vi "Aircraft Main.vi"(8 "error out":errorcluster, 11 "Aircraft Index":u8) -> (0 "error out 2":errorcluster)   [LabVIEW 2014]
uses:
  Application Support/Stop Button/SubVI/Get Stop Button Status.vi
  MAVLink/Commands/MAV_CMD Sub VI/MAV_CMD_COMPONENT_ARM_DISARM.vi
  Controls/Aircraft State.ctl
  Joystick/FGVs/Joystick Input/Method VIs/Get Joystick Input.vi
  Aircraft Information/Sub VI/Get Aircraft System Status.vi
  Aircraft Information/Sub VI/Set Aircraft System Status.vi
  Aircraft Information/Controls/Aircraft RC Data.ctl
  Aircraft Information/Controls/Aircraft Attitude Data.ctl
  Aircraft Information/Controls/Base Mode.ctl
  Aircraft Information/Controls/Drone Information.ctl
  Aircraft Information/Controls/Aircraft Mode.ctl
  Aircraft Information/Controls/Aircraft Sensor Status Data.ctl
  GUI Design/Indicators/Status LED.ctl
  GUI Design/Indicators/Sensor Status LED CLuster.ctl
  Controls/Telemetry Connection Type.ctl
panel:
  in  "Altitude (m)":sgl
  in  "Takeoff":bool
  in  "Main Tab":T1(tab)
  in  "Aircraft State":T2=enum."Initialise"
  out "Aircraft Att Data Out":T3
  out "Aircraft RC Data Out":T4
  out "Control Mode":T5=enum."Stabalise"
  out "Armed/Disarmed":bool
  in  "param_id":string
  in  "Request Param":bool
  in  "Get Message":bool
  in  "Message Rate (hz)":u16=5
  in  "start_stop":bool
  in  "req_stream_id":T6(ring)
  in  "Aircraft Update Rate (Hz)":dbl=30.0
  in  "Release Control":bool
  out "TX Queue State":i32(slide) scale=0.0..50.0
  out "RX Queue State":i32(slide) scale=0.0..50.0
  out "System Status Out":T7 {"Communication Drop Rate (%)" scale=0.0..100.0; "Battery Remaining (%)" scale=0.0..100.0; "CPU Load (%)" scale=0.0..100.0}
  out "Status text":string
  in  "Clear Status Text":bool
  in  "ARM/DISARM":bool
  out "Drone Information Out":T10={"Heart Beat"=FALSE, "Aircraft ID"=0, "Downlink Port"="", "Tag ID"="", "System Status"="", "Base Mode"={"Custom Mode"=FALSE, "Test Enabled"=FALSE, "Autonomous Mode"=FALSE, "Guided Mode"=FALSE, "Stabilization Enabled"=FALSE, "HIL Enabled"=FALSE, "Manual Mode"=FALSE, "Arm"=FALSE}, "Armed/Disarmed"=FALSE, "Battery Voltage"=0.0, "Control Mode"=enum."Stabalise", "Initialisation"=0, "Heart Beat Status"=FALSE, "Uplink Port"="", "UDP connection ID"=refnum, "Connection Type"=enum."Serial", "Mode"="", "UDP IP Address"="", "Mission Uploaded"=FALSE} {"Initialisation" scale=0.0..100.0}
  out "Initialisation Progress":u8(slide) scale=0.0..100.0
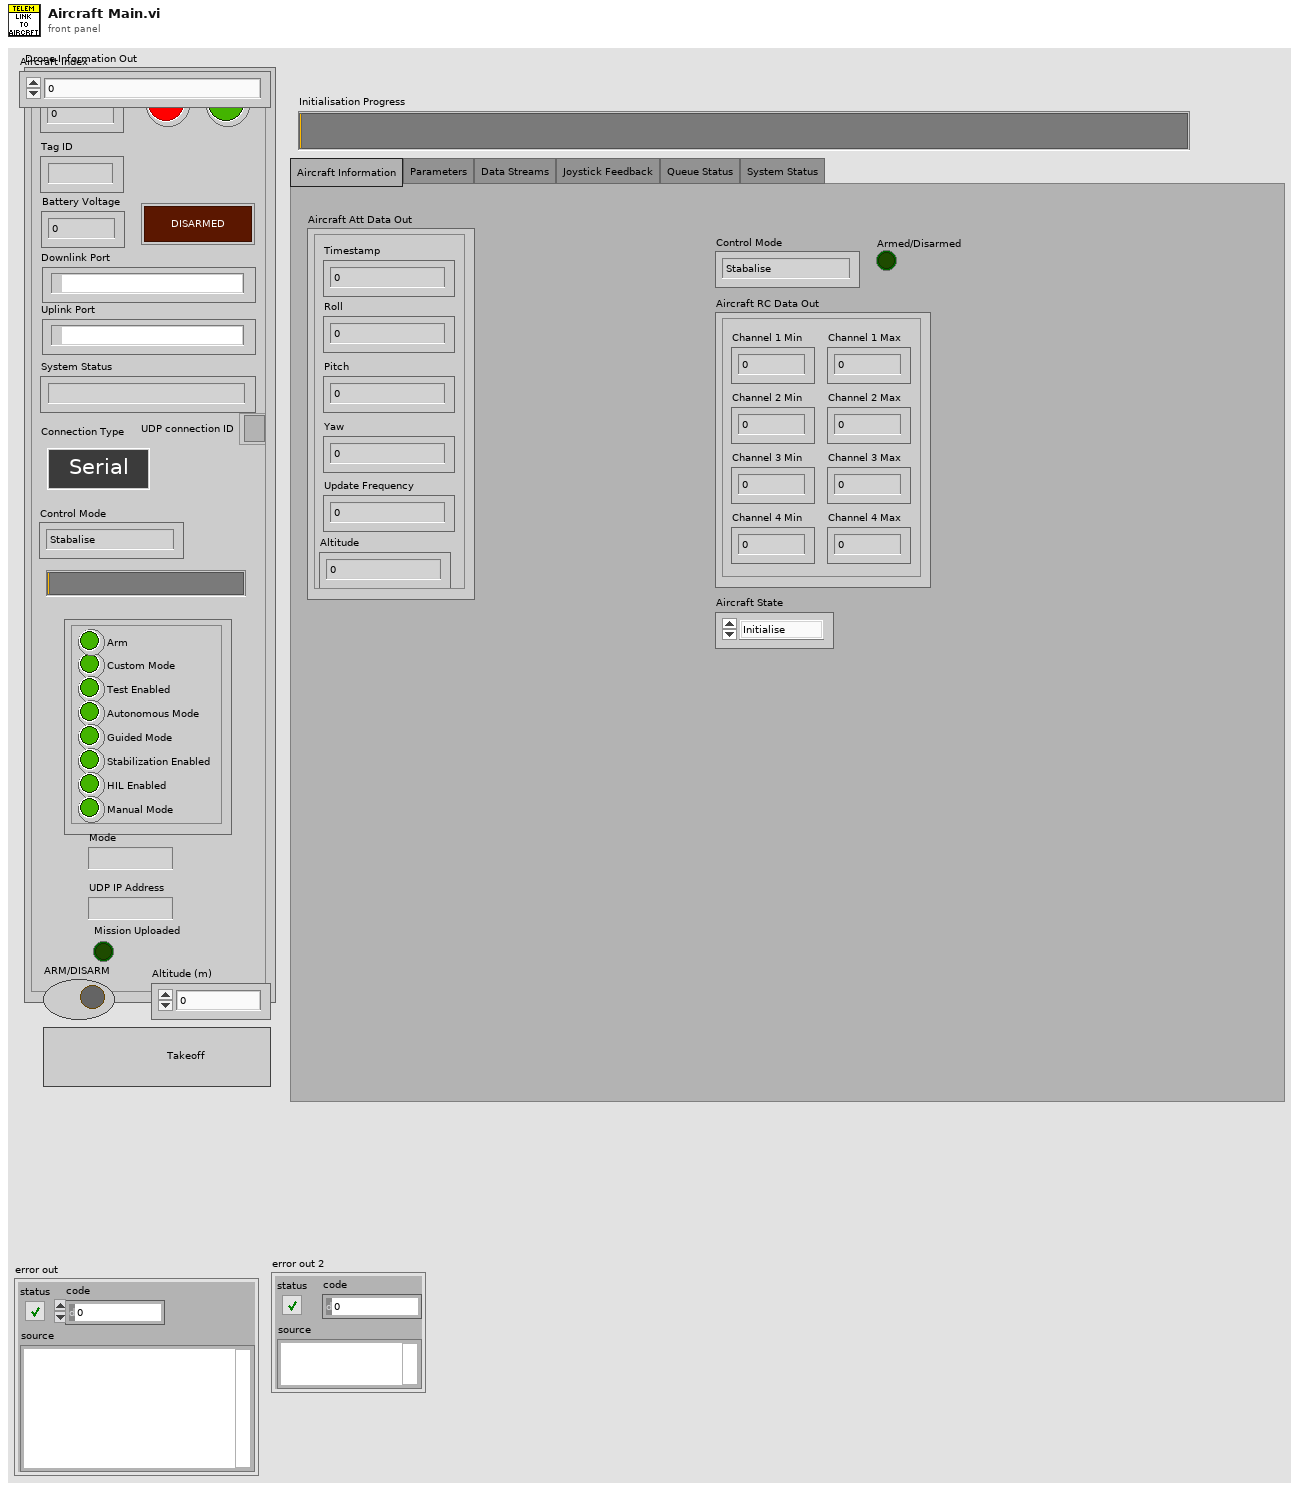
[diagram p1: front panel]
types:
  T1 = enum32{"Aircraft Information", "Parameters", "Data Streams", "Joystick Feedback", "Queue Status", "System Status"}
  T2 = typedef "Aircraft State.ctl" = enum16{"Connected", "Initialise", "Disconnected"}
  T3 = typedef "Aircraft Attitude Data.ctl" = cluster{"Roll":sgl, "Pitch":sgl, "Yaw":sgl, "Timestamp":u32, "Update Frequency":dbl, "Altitude":sgl}
  T4 = typedef "Aircraft RC Data.ctl" = cluster{"Channel 1 Min":i16, "Channel 1 Max":i16, "Channel 2 Min":i16, "Channel 2 Max":i16, "Channel 3 Min":i16, "Channel 3 Max":i16, "Channel 4 Min":i16, "Channel 4 Max":i16}
  T5 = typedef "Aircraft Mode.ctl" = enum16{"Loiter", "Stabalise", "Failsafe", "Emergency Stop"}
  T6 = enum16{"ALL", "RAW_SENSORS", "EXTENDED_STATUS", "RC_CHANNELS", "RAW_CONTROLLER", "POSITION", "EXTRA1", "EXTRA2", "EXTRA3"}
  T7 = typedef "Aircraft Sensor Status Data.ctl" = cluster{"Sensor Status":T8, "CPU Load (%)":dbl, "Battery Voltage (V)":dbl, "Battery Current (A)":dbl, "Battery Remaining (%)":dbl, "Communication Drop Rate (%)":dbl, "Communication Errors (%)":dbl, "Status text":string}
  T8 = typedef "Sensor Status LED CLuster.ctl" = cluster{"3D Gyro":u32, "3D Accel":u32, "3D Mag":u32, "Abs. Pressure":u32, "Diff. Pressure":u32, "GPS":T9, "Optical Flow":u32, "Vision Position":u32, "Laser Position":u32, "External Ground Truth":u32, "Angular Rate Control":u32, "Attitude Stabilisation":u32, "Yaw Position":u32, "Z Altitude Control":u32, "XY Position Control":u32, "Motor Outputs":u32, "RC Receiver":u32, "3D Gyro 2":u32, "3D Accel 2":u32, "3D Mag 2":u32, "Geofence":u32, "AHRS":u32, "Terrain":u32}
  T9 = typedef "Status LED.ctl" = u32
  T10 = typedef "Drone Information.ctl" = cluster{"Heart Beat":bool, "Aircraft ID":u8, "Downlink Port":refnum<visa-resource-name>, "Tag ID":string, "System Status":string, "Base Mode":T11, "Armed/Disarmed":bool, "Battery Voltage":dbl, "Control Mode":T5, "Initialisation":u8, "Heart Beat Status":bool, "Uplink Port":refnum<visa-resource-name>, "UDP connection ID":refnum<k16>, "Connection Type":T12, "Mode":string, "UDP IP Address":string, "Mission Uploaded":bool}
  T11 = typedef "Base Mode.ctl" = cluster{"Custom Mode":bool, "Test Enabled":bool, "Autonomous Mode":bool, "Guided Mode":bool, "Stabilization Enabled":bool, "HIL Enabled":bool, "Manual Mode":bool, "Arm":bool}
  T12 = typedef "Telemetry Connection Type.ctl" = enum16{"Serial", "UDP", "TCP"}
  T13 = typedef "Joystick Input.ctl" = cluster{"Roll (%)":dbl, "Pitch (%)":dbl, "Yaw (%)":dbl, "Throttle (%)":dbl, "Brake":bool, "Emergency Stop":bool, "Arm":bool, "Disarm":bool}
  T14 = cluster{"req_message_rate":u16, "target_system":u8, "target_component":u8, "req_stream_id":enum16{"ALL", "RAW_SENSORS", "EXTENDED_STATUS", "RC_CHANNELS", "RAW_CONTROLLER", "POSITION", "EXTRA1", "EXTRA2", "EXTRA3"}, "start_stop":bool}
  T15 = cluster{"chan1_raw":u16, "chan2_raw":u16, "chan3_raw":u16, "chan4_raw":u16, "chan5_raw":u16, "chan6_raw":u16, "chan7_raw":u16, "chan8_raw":u16, "target_system":u8, "target_component":u8}
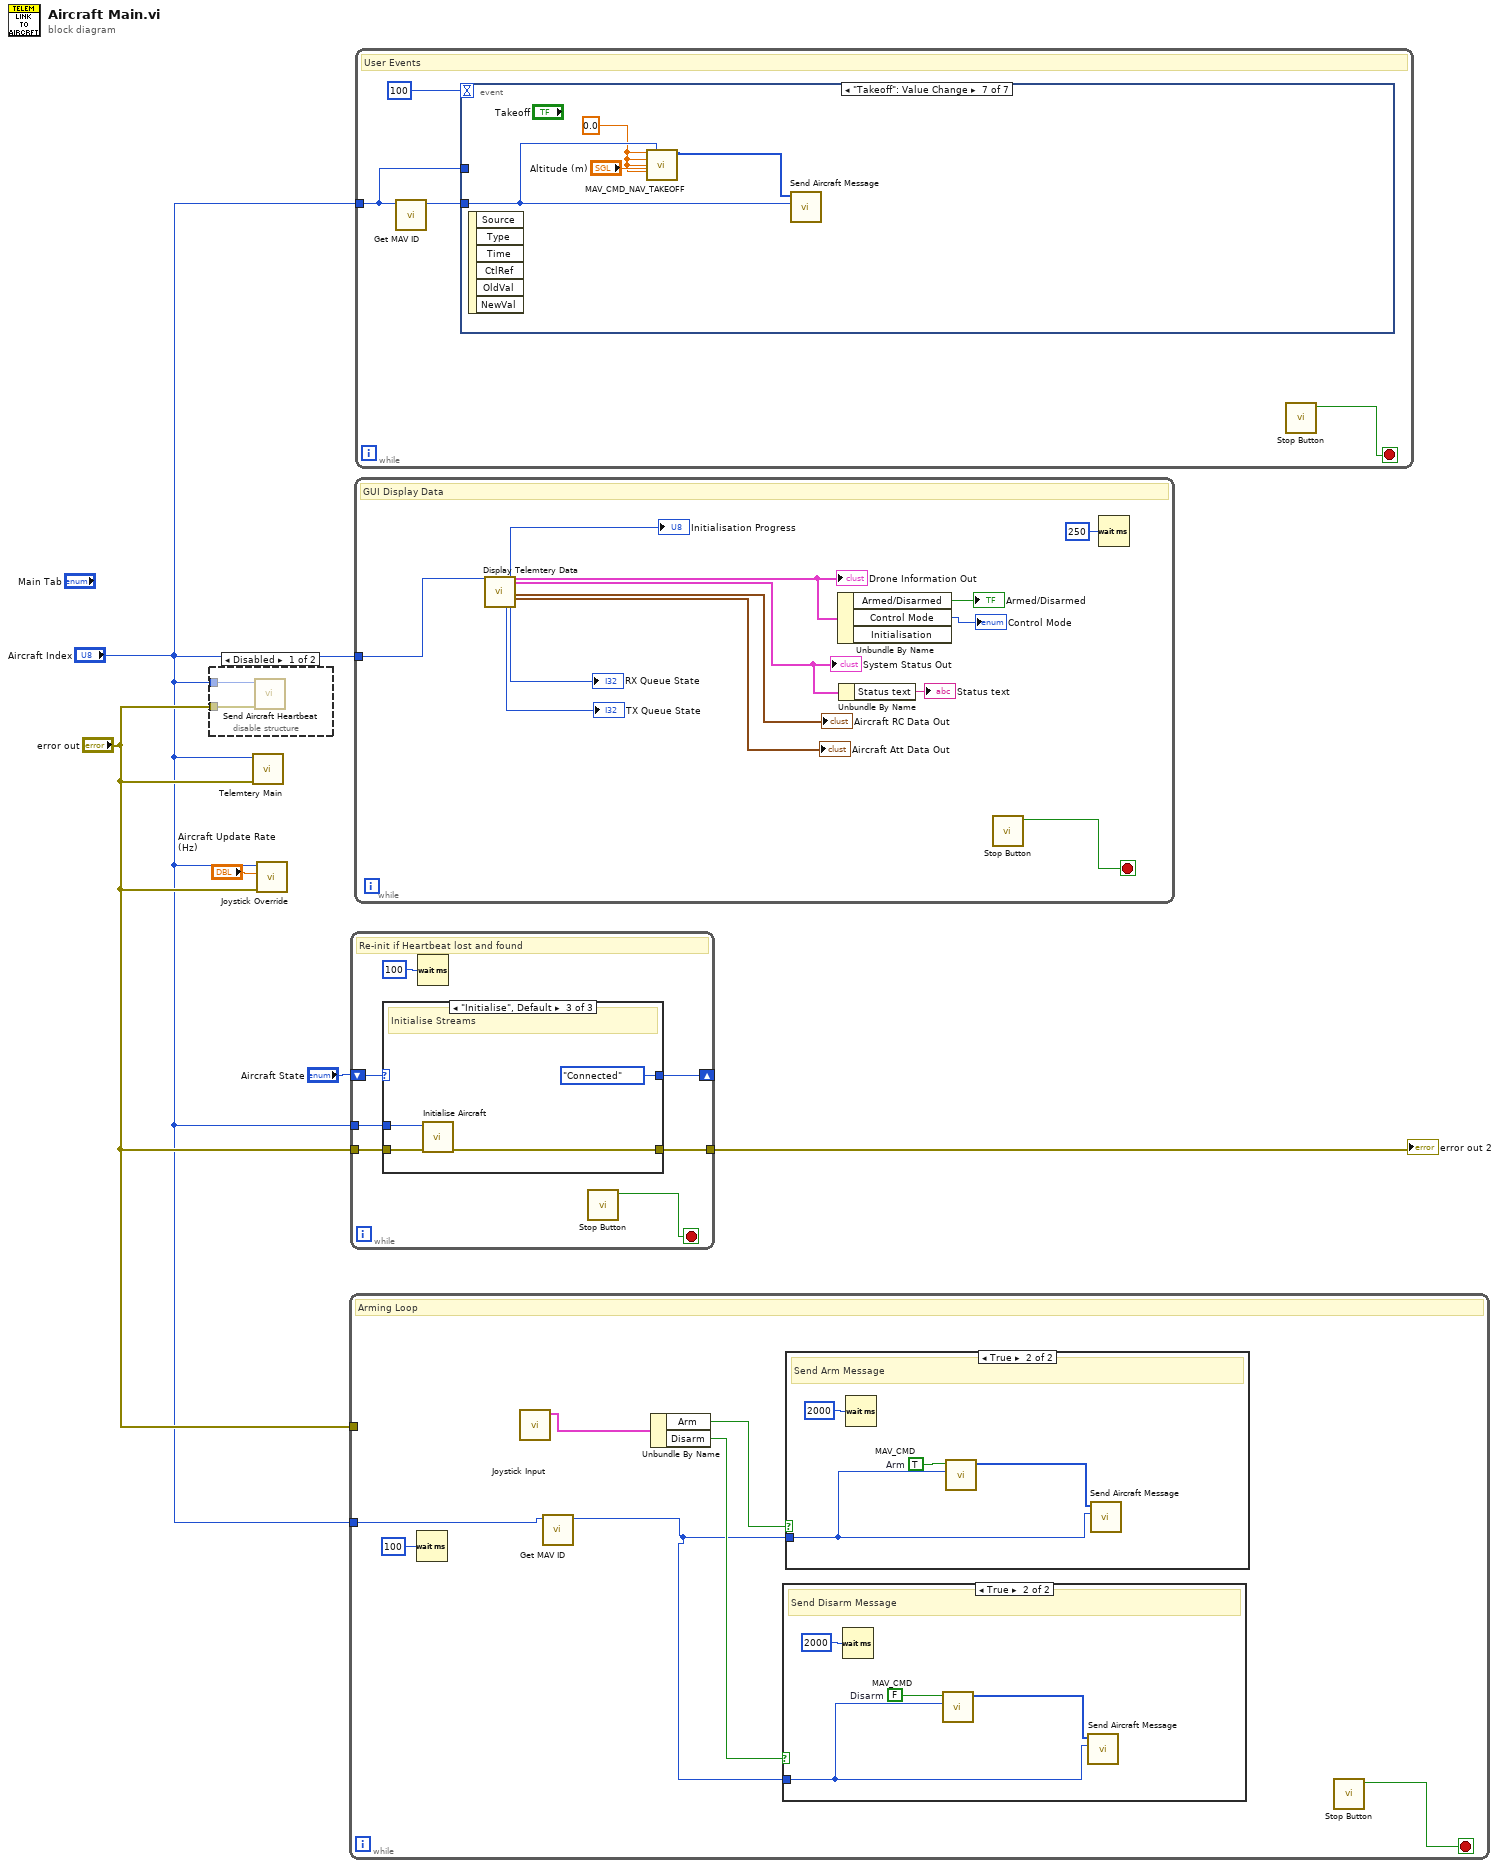
[diagram p0: block diagram]
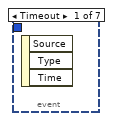
[diagram p5: hidden frame]
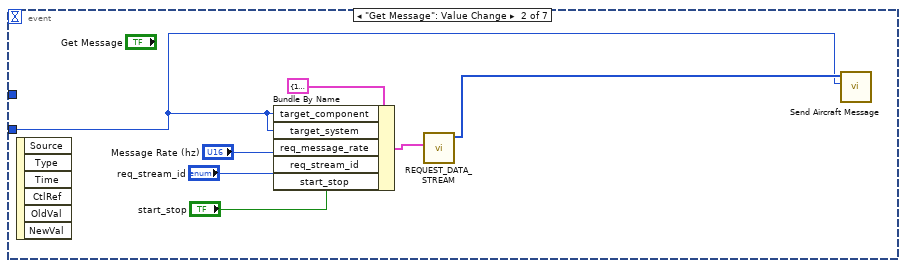
[diagram p6: hidden frame]
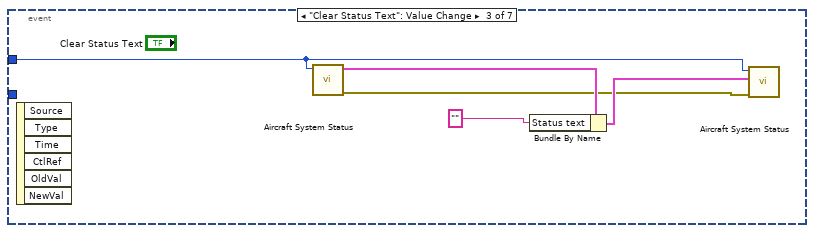
[diagram p7: hidden frame]
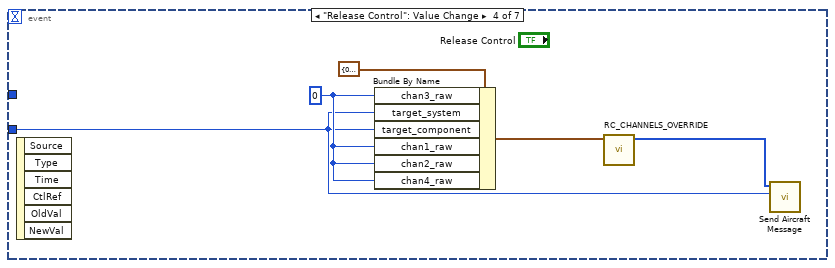
[diagram p8: hidden frame]
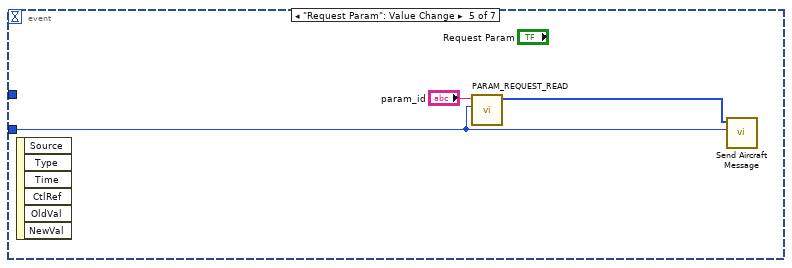
[diagram p9: hidden frame]
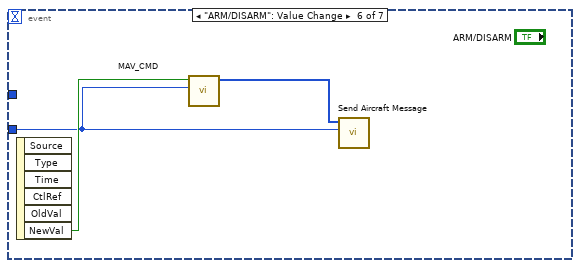
[diagram p10: hidden frame]
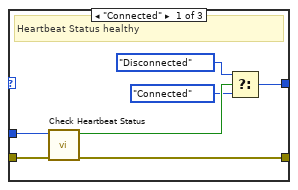
[diagram p11: hidden frame]
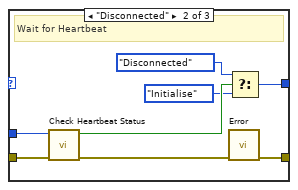
[diagram p12: hidden frame]
diagram:
  n1 = disable-structure shown="Disabled" {
    disable-tunnel: "error out" -> [w7 _]
    disable-tunnel: "Aircraft Index" -> [w6 _]
    frame Disabled {
      n2 = call "Send Aircraft Heartbeat.vi"("error in (no error)"=w7, "Aircraft ID"=w6) -> ()  [unwired: 10 in]
    }
    frame Enabled {
    }
  }
  n3 = call "Telemtery Main.vi"("error IN"="error out", "Aircraft Index"="Aircraft Index") -> ()  [unwired: 10 in]
  n4 = call "Joystick Override.vi"("error in (no error)"="error out", "Aircraft Update Rate (Hz)"="Aircraft Update Rate (Hz)", "Aircraft ID"="Aircraft Index") -> ()  [unwired: 9 in]
  n5 = while {
    tunnel: "Aircraft Index" -> [w12]
    tunnel: "error out" -> [_]
    stop <- w13 stop-if-true
    # "Arming Loop"
    n6 = Wait (ms)(milliseconds to wait=u32 100) -> ()  [unwired: 1 out]
    n7 = call-poly "Joystick Input.vi"() -> ("Joystick Input Out"=w11:T13)  [unwired: 11 in]
    n8 = call "Get MAV ID.vi"("Aircraft Index"=w12) -> ("Aircraft ID"=w8:u8)  [unwired: 9 in, 1 out]
    n9 = Unbundle By Name(w11) -> ("Arm"=w9:bool, "Disarm"=w10:bool)
    n10 = case shown="True" w10 {
      tunnel: w8 -> [_ w19]
      frame False {
      }
      frame True {
        w22 = FALSE  # Disarm
        # "Send Disarm Message"
        n11 = Wait (ms)(milliseconds to wait=u32 2000) -> ()  [unwired: 1 out]
        n12 = call-poly "MAV_CMD.vi"("Target System and Target Component"=w19, "ARM(T)/DISARM(F)"=w22) -> ("MAVLink Message"=w21:u8[])  [unwired: 9 in]
        n13 = call "Send Aircraft Message.vi"("Aircraft ID"=w19, "MAVLink Message"=w21) -> ()  [unwired: 9 in, 1 out]
      }
    }
    n14 = case shown="True" w9 {
      tunnel: w8 -> [_ w15]
      frame False {
      }
      frame True {
        w18 = TRUE  # Arm
        # "Send Arm Message"
        n15 = Wait (ms)(milliseconds to wait=u32 2000) -> ()  [unwired: 1 out]
        n16 = call-poly "MAV_CMD.vi"("Target System and Target Component"=w15, "ARM(T)/DISARM(F)"=w18) -> ("MAVLink Message"=w17:u8[])  [unwired: 9 in]
        n17 = call "Send Aircraft Message.vi"("Aircraft ID"=w15, "MAVLink Message"=w17) -> ()  [unwired: 9 in, 1 out]
      }
    }
    n18 = call-poly "Stop Button.vi"() -> ("Stop ButtonOut"=w13:bool)  [unwired: 10 in, 1 out]
  }
  n19 = while {
    tunnel: "error out" -> [w25]
    tunnel: "Aircraft Index" -> [w29]
    shift-right: [w26] -> _
    shift-left: "Aircraft State" -> [w27]
    tunnel: [w23] -> w3
    stop <- w28 stop-if-true
    # "Re-init if Heartbeat lost and found"
    n20 = case shown="\"Initialise\", Default" w27 {
      tunnel: w25 -> [w36 w43 w47]
      tunnel: w29 -> [w35 w42 w46]
      tunnel: [w30 w38 Aircraft_State."Connected" ("Aircraft State")] -> w26
      tunnel: [w31 w37 w45] -> w23
      frame "Connected" {
        # "Heartbeat Status healthy"
        n21 = call "Check Heartbeat Status.vi"("Error In"=w36, "Aircraft ID"=w35) -> ("Error Out"=w31:errorcluster, "Heartbeat Lost"=w34:bool)  [unwired: 8 in]
        n22 = Select(t=Aircraft_State."Disconnected" ("Aircraft State"), s=w34, f=Aircraft_State."Connected") -> (s? t:f=w30:T2)
      }
      frame "Disconnected" {
        # "Wait for Heartbeat"
        n23 = call "Check Heartbeat Status.vi"("Error In"=w43, "Aircraft ID"=w42) -> ("Error Out"=w41:errorcluster, "Heartbeat Lost"=w44:bool)  [unwired: 8 in]
        n24 = call "Error.vi"("Error In"=w41) -> ("Error Out"=w37:errorcluster)  [unwired: 10 in]
        n25 = Select(t=Aircraft_State."Disconnected", s=w44, f=Aircraft_State."Initialise" ("Aircraft State")) -> (s? t:f=w38:T2)
      }
      frame "Initialise", Default {
        # "Initialise Streams"
        n26 = call "Initialise Aircraft.vi"("error IO"=w47, "Aircraft ID"=w46) -> ("error out"=w45:errorcluster)  [unwired: 9 in]
      }
    }
    n27 = Wait (ms)(milliseconds to wait=u32 100) -> ()  [unwired: 1 out]
    n28 = call-poly "Stop Button.vi"() -> ("Stop ButtonOut"=w28:bool)  [unwired: 10 in, 1 out]
  }
  "error out 2" <- w3
  n29 = while {
    tunnel: "Aircraft Index" -> [w59]
    stop <- w61 stop-if-true
    # "GUI Display Data"
    n30 = call "Display Telemtery Data.vi"("Instance Details"=w59) -> ("TX Queue State"=→"TX Queue State":i32, "Initialisation Progress"=→"Initialisation Progress":u8, "RX Queue State"=→"RX Queue State":i32, "Drone Information Out"=w57:T10, "System Status Out"=w53:T7, "Aircraft RC Data Out"=→"Aircraft RC Data Out":T4, "Aircraft Att Data Out"=→"Aircraft Att Data Out":T3)  [unwired: 17 in, 3 out]
    "System Status Out" <- w53
    "Drone Information Out" <- w57
    n31 = Unbundle By Name(w57) -> ("Armed/Disarmed"=→"Armed/Disarmed":bool, "Control Mode"=→"Control Mode":T5)  [unwired: 1 out]
    n32 = Unbundle By Name(w53) -> ("Status text"=→"Status text":string)
    n33 = call-poly "Stop Button.vi"() -> ("Stop ButtonOut"=w61:bool)  [unwired: 10 in, 1 out]
    n34 = Wait (ms)(milliseconds to wait=u32 250) -> ()  [unwired: 1 out]
  }
  n35 = while {
    tunnel: "Aircraft Index" -> [w62]
    stop <- w64 stop-if-true
    # "User Events"
    n36 = call "Get MAV ID.vi"("Aircraft Index"=w62) -> ("Aircraft ID"=w63:u8)  [unwired: 9 in, 1 out]
    n37 = event shown="[6] \"Takeoff\": Value Change" {
      selector: _ -> [_ _ _ _ _ _ _]
      dyn-events: _ -> [_ _ _ _ _ _ _]
      timeout: 100 -> [_ _ _ _ _ _ _]
      tunnel: w63 -> [_ w70 _ w78 w83 w86 w91]
      tunnel: w62 -> [_ _ w73 _ _ _ _]
      event Timeout {
        n38 = event-data() -> ()  [unwired: 1 in, 3 out]
      }
      event "Get Message": Value Change {
        n39 = event-data() -> ()  [unwired: 1 in, 6 out]
        n40 = Bundle By Name(cluster=T14 {"req_message_rate"=10, "target_system"=0, "target_component"=0, "req_stream_id"=enum."ALL", "start_stop"=FALSE} ("Payload"), "target_component"=w70, "target_system"=w70, "req_message_rate"="Message Rate (hz)", "req_stream_id"="req_stream_id", "start_stop"="start_stop") -> (w66:T14)
        n41 = call "REQUEST_DATA_STREAM.vi"("Payload"=w66) -> ("MAVLink MSG"=w72:u8[])  [unwired: 10 in]
        n42 = call "Send Aircraft Message.vi"("Aircraft ID"=w70, "MAVLink Message"=w72) -> ()  [unwired: 9 in, 1 out]
      }
      event "Clear Status Text": Value Change {
        n43 = event-data() -> ()  [unwired: 1 in, 6 out]
        n44 = call-poly "Aircraft System Status.vi"("Aircraft ID"=w73) -> ("Error Out"=w74:errorcluster, "System Status Out"=w77:T7)  [unwired: 9 in]
        n45 = Bundle By Name(cluster=w77, "Status text"="") -> (w75:T7)
        n46 = call-poly "Aircraft System Status.vi"("Error In"=w74, "System Status In"=w75, "Aircraft ID"=w73) -> ()  [unwired: 8 in, 1 out]
      }
      event "Release Control": Value Change {
        w80 = u16 0 ("chan3_raw")
        n47 = event-data() -> ()  [unwired: 1 in, 6 out]
        n48 = Bundle By Name(cluster=T15 {"chan1_raw"=0, "chan2_raw"=0, "chan3_raw"=0, "chan4_raw"=0, "chan5_raw"=0, "chan6_raw"=0, "chan7_raw"=0, "chan8_raw"=0, "target_system"=0, "target_component"=0} ("Payload"), "chan3_raw"=w80, "target_system"=w78, "target_component"=w78, "chan1_raw"=w80, "chan2_raw"=w80, "chan4_raw"=w80) -> (w82:T15)
        n49 = call "RC_CHANNELS_OVERRIDE.vi"("Payload"=w82) -> ("MAVLink Message"=w79:u8[])  [unwired: 10 in]
        n50 = call "Send Aircraft Message.vi"("Aircraft ID"=w78, "MAVLink Message"=w79) -> ()  [unwired: 9 in, 1 out]
      }
      event "Request Param": Value Change {
        n51 = event-data() -> ()  [unwired: 1 in, 6 out]
        n52 = call "PARAM_REQUEST_READ.vi"("Target System and Target Component"=w83, "param_id"="param_id") -> ("MAVLink Message"=w84:u8[])  [unwired: 9 in]
        n53 = call "Send Aircraft Message.vi"("Aircraft ID"=w83, "MAVLink Message"=w84) -> ()  [unwired: 9 in, 1 out]
      }
      event "ARM/DISARM": Value Change {
        n54 = event-data() -> ("NewVal"=w88:bool)  [unwired: 1 in, 5 out]
        n55 = call-poly "MAV_CMD.vi"("Target System and Target Component"=w86, "ARM(T)/DISARM(F)"=w88) -> ("MAVLink Message"=w87:u8[])  [unwired: 9 in]
        n56 = call "Send Aircraft Message.vi"("Aircraft ID"=w86, "MAVLink Message"=w87) -> ()  [unwired: 9 in, 1 out]
      }
      event "Takeoff": Value Change {
        w89 = sgl 0.0 ("Yaw Angle")
        n57 = event-data() -> ()  [unwired: 1 in, 6 out]
        n58 = call "MAV_CMD_NAV_TAKEOFF.vi"("Minimum Pitch"=w89, "Aircraft ID"=w91, "Yaw Angle"=w89, "Latitude"=w89, "Longitude"=w89, "Altitude (m)"="Altitude (m)") -> ("MAVLink Message"=w92:u8[])  [unwired: 9 in]
        n59 = call "Send Aircraft Message.vi"("Aircraft ID"=w91, "MAVLink Message"=w92) -> ()  [unwired: 9 in, 1 out]
      }
    }
    n60 = call-poly "Stop Button.vi"() -> ("Stop ButtonOut"=w64:bool)  [unwired: 10 in, 1 out]
  }
